vi "Serial LabVIEW to Arduino.vi"() -> ()   [LabVIEW 2014]
uses:
  <vilib>/Instr/_visa.llb/VISA Configure Serial Port (Instr).vi
panel:
  in  "Write?":bool
  in  "write buffer":string
  out "Bytes to Read":u32
  out "read buffer":string
  in  "stop":bool
  in  "baud rate (9600)":u32=19200
  in  "VISA resource name":refnum<visa-resource-name>="COM6"
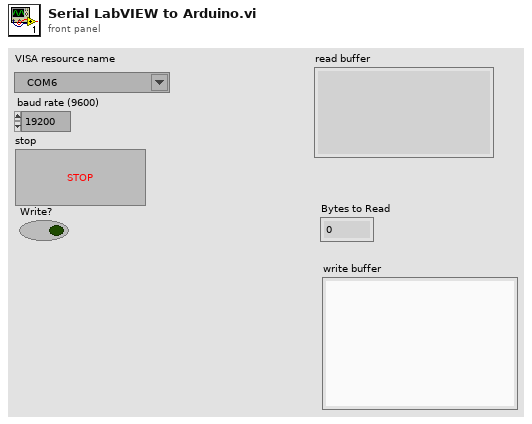
[diagram p1: front panel]
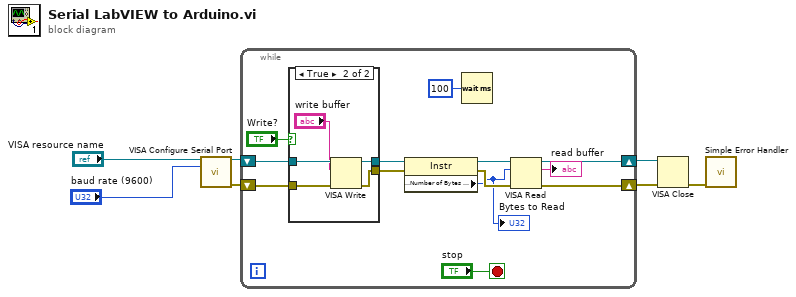
[diagram p0: block diagram]
diagram:
  n1 = call-poly "VISA Configure Serial Port"("VISA resource name"="VISA resource name", "baud rate (9600)"="baud rate (9600)") -> ("VISA resource name out"=w7:refnum<visa-resource-name>, "error out"=w6:errorcluster)  [unwired: 12 in]
  n2 = while {
    shift-right: [w19] -> w3
    shift-left: w7 -> [w12]
    shift-right: [w17] -> w2
    shift-left: w6 -> [w10]
    stop <- "stop" stop-if-true
    n3 = case shown="True" "Write?" {
      tunnel: w12 -> [w22 w27]
      tunnel: [w22 w26] -> w11
      tunnel: w10 -> [w21 w25]
      tunnel: [w21 w24] -> w9
      frame False {
      }
      frame True {
        n4 = VISA Write(VISA resource name=w27, write buffer="write buffer", error in (no error)=w25) -> (VISA resource name out=w26:refnum<visa-resource-name>, error out=w24:errorcluster)  [unwired: 1 out]
      }
    }
    n5 = property class="Instr"(reference=w11, error in=w9) -> (reference out=w20:refnum<visa-resource-name>, error out=w18:errorcluster, "Serial Settings:Number of Bytes at Serial Port"=w13:u32)
    "Bytes to Read" <- w13
    n6 = Wait (ms)(milliseconds to wait=u32 100) -> ()  [unwired: 1 out]
    n7 = VISA Read(VISA resource name=w20, byte count=w13, error in (no error)=w18) -> (VISA resource name out=w19:refnum<visa-resource-name>, read buffer=→"read buffer":string, error out=w17:errorcluster)  [unwired: 1 out]
  }
  n8 = VISA Close(VISA resource name=w3, error in (no error)=w2) -> (error out=w1:errorcluster)
  n9 = call <vilib>:"Simple Error Handler.vi"("error in (no error)"=w1) -> ()  [unwired: 4 in, 5 out]
